vi "Stop.vi"(8 "error in (no error)":errorcluster, 11 "Electrophysiology in":refnum<class "AcquireTraces.lvclass">) -> (0 "error out":errorcluster, 3 "Electrophysiology out":refnum<class "AcquireTraces.lvclass">)   [LabVIEW 2014, in "AcquireTraces.lvclass"]
uses:
  AcquireTraces.lvclass
  AcquireTraces.lvclass/AcquireTraces.ctl
  HDF5Tools/LabView/HDF5Tools.lvlib
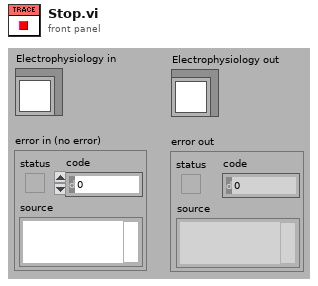
[diagram p1: front panel]
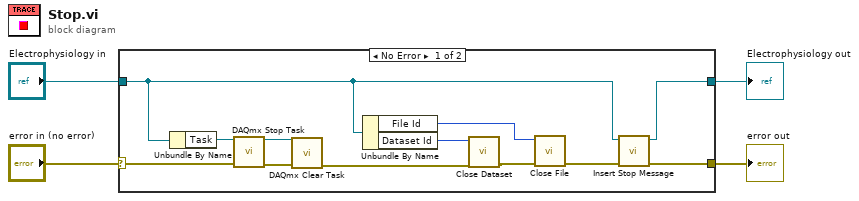
[diagram p0: block diagram]
diagram:
  n1 = case shown="No Error" "error in (no error)" {
    selector: "error in (no error)" -> [w13 w18]
    tunnel: [w7 w18] -> w3
    tunnel: [w5 w17] -> w1
    tunnel: "Electrophysiology in" -> [w6 w17]
    frame No Error {
      n2 = Unbundle By Name(w6) -> ("Task"=w14:refnum<k21>)
      n3 = call <vilib>:"DAQmx Stop Task.vi"("task/channels in"=w14, "error in"=w13) -> ("task out"=w16:refnum<k21>, "error out"=w15:errorcluster)  [unwired: 12 in]
      n4 = call <vilib>:"DAQmx Clear Task.vi"("task in"=w16, "error in"=w15) -> ("error out"=w9:errorcluster)  [unwired: 13 in]
      n5 = Unbundle By Name(w6) -> ("File Id"=w12:u64, "Dataset Id"=w11:u64)
      n6 = call "Close Dataset.vi"("error in (no error)"=w9, "dataset_id"=w11) -> ("error out"=w10:errorcluster)  [unwired: 9 in]
      n7 = call "Close File.vi"("error in (no error)"=w10, "file_id"=w12) -> ("error out"=w8:errorcluster)  [unwired: 9 in]
      n8 = call-dynamic "Insert Stop Message.vi"("error in (no error)"=w8, "AcquireTraces in"=w6) -> ("error out"=w7:errorcluster, "AcquireTraces out"=w5:refnum<class "AcquireTraces.lvclass">)  [unwired: 8 in]
    }
    frame Error {
    }
  }
  "error out" <- w3
  "Electrophysiology out" <- w1
